vi "Startup Motor.vi"(8 "error in (no error)":errorcluster, 10 "Motor Controller":refnum<class "Motor Controller.lvclass">, 11 "TopLevel in":refnum<class "TopLevel.lvclass">) -> (0 "error out":errorcluster)   [LabVIEW 2022 SP3, in "Motor Controller.lvclass"]
uses:
  Motor Controller.lvclass
  TopLevel/TopLevel.lvclass
  Motor Controller_Process.vi
panel:
  out "timed out?":bool
  out "sync from process?":bool
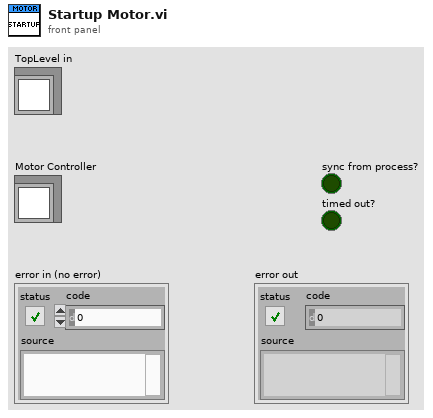
[diagram p1: front panel]
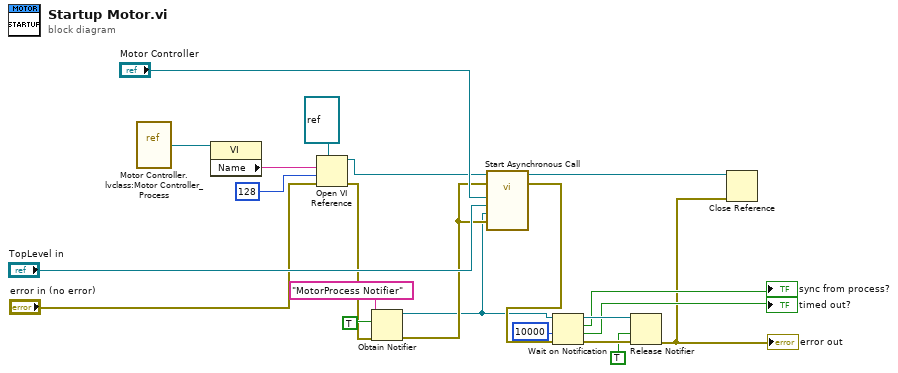
[diagram p0: block diagram]
diagram:
  n1 = vi-ref "Motor Controller.lvclass:Motor Controller_Process.vi"() -> (w14:refnum<vi>)
  n2 = property class="VI"(reference=w14) -> ("Name"=w15:string)  [unwired: 1 in, 2 out]
  n3 = Open VI Reference(type specifier VI Refnum (for type only)=refnum<vi> refnum, vi path=w15, options=128, error in (no error)="error in (no error)") -> (vi reference=w18:refnum<vi>, error out=w11:errorcluster)  [unwired: 2 in]
  n4 = Obtain Notifier(name (unnamed)="MotorProcess Notifier", notification data type=TRUE, error in (no error)=w11) -> (notifier out=w1:refnum<notifier>, error out=w10:errorcluster)  [unwired: 1 in, 1 out]
  n5 = call-by-ref "Start Asynchronous Call"(reference=w18, error in=w10, "error in"=w10, "Process Sync"=w1, "TopLevel"="TopLevel in", "Motor Controller in"="Motor Controller") -> (reference out=w19:refnum<vi>, error out=w3:errorcluster)  [unwired: 7 in, 1 out]
  n6 = Wait on Notification(notifier=w1, timeout in ms (-1)=10000, error in (no error)=w3) -> (notifier out=w7:refnum<notifier>, notification=→"sync from process?":bool, timed out?=→"timed out?":bool, error out=w8:errorcluster)  [unwired: 1 in]
  n7 = Release Notifier(notifier=w7, force destroy? (F)=TRUE, error in (no error)=w8) -> (error out=w2:errorcluster)  [unwired: 2 out]
  "error out" <- w2
  n8 = Close Reference(reference=w19, error in (no error)=w2) -> ()  [unwired: 1 out]
